vi "Terminal-Modbus-ReadRegisters.vi"(8 "error in (no error)":errorcluster caption="错误输入（无错误）", 10 "簇":T1, 11 "ModbusMsgQRef":refnum<queue>) -> (0 "error out":errorcluster caption="错误输出")   [LabVIEW 2014]
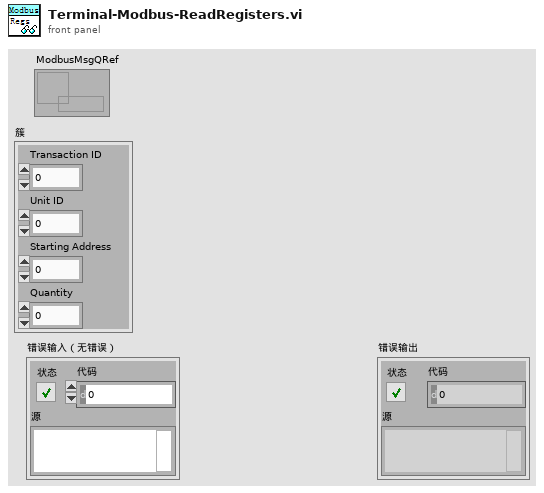
[diagram p1: front panel]
types:
  T1 = cluster{"Transaction ID":u16, "Unit ID":u8, "Starting Address":u16, "Quantity":u16}
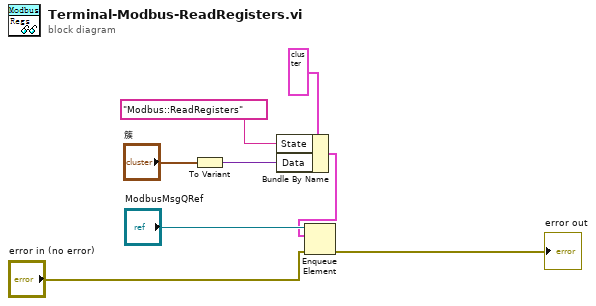
[diagram p0: block diagram]
diagram:
  n1 = To Variant(anything="簇") -> (Variant=w3:variant)
  n2 = Bundle By Name(cluster=cluster{"Data":variant, "State":string} {"Data"=variant, "State"=""} ("元素"), "State"="Modbus::ReadRegisters", "Data"=w3) -> (w1:cluster{"Data":variant, "State":string})
  n3 = Enqueue Element(queue="ModbusMsgQRef", element=w1, error in (no error)="error in (no error)") -> (error out=→"error out":errorcluster)  [unwired: 1 in, 2 out]
